vi "Get My Computer Build Spec Children__icon_lib_labview_project_api.vi"(8 "error in (no error)":errorcluster, 11 "Project Reference":refnum<vi>) -> (0 "error out":errorcluster, 2 "Children[]":refnum<vi>[](array[refnum]), 3 "Project Reference Dup":refnum<vi>)   [LabVIEW 2016, in "LabVIEW Project API__icon_lib_labview_project_api.lvlib"]
doc: "Given a Project Path, this VI returns all the Build Spec Children references for the My Computer Target.\n\n<b>Author:</b> JG\n\n<b>ICON Technologies Pty Ltd</b>\nCopyright (C) 1990-2009\nAll Rights Reserved"
uses:
  LabVIEW Project API__icon_lib_labview_project_api.lvlib
panel:
  # "Output"
  # "Input"
  # "ICON Technologies Pty Ltd\nCopyright (C) 1990-2009\nAll Rights Reserved"
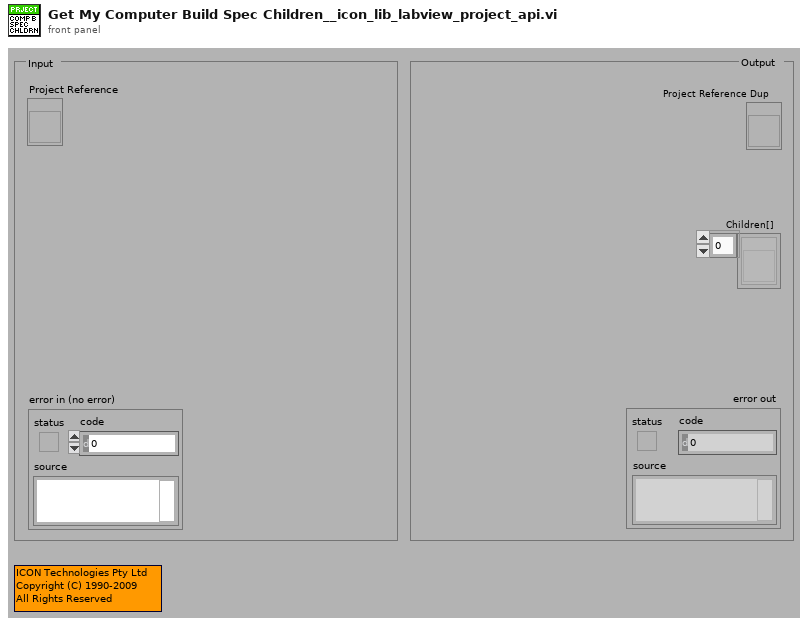
[diagram p1: front panel]
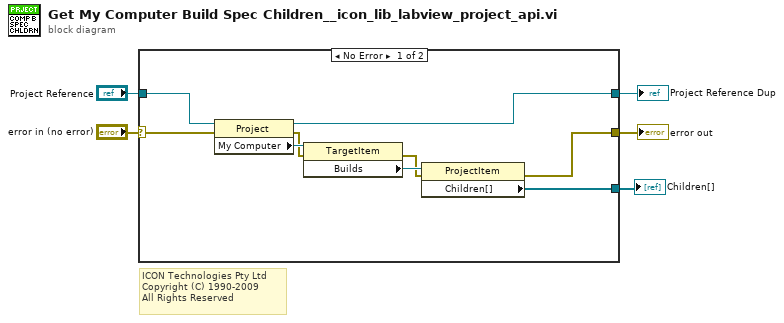
[diagram p0: block diagram]
diagram:
  # "ICON Technologies Pty Ltd\nCopyright (C) 1990-2009\nAll Rights Reserved"
  n1 = case shown="No Error" "error in (no error)" {
    selector: "error in (no error)" -> [w6 w16]
    tunnel: [w8 w16] -> w4
    tunnel: [w10 _] -> w3
    tunnel: [w9 w15] -> w2
    tunnel: "Project Reference" -> [w7 w15]
    frame No Error {
      n2 = property class="Project"(reference=w7, error in=w6) -> (reference out=w9:refnum<vi>, error out=w13:errorcluster, "My Computer"=w14:refnum<vi>)
      n3 = property class="TargetItem"(reference=w14, error in=w13) -> (error out=w11:errorcluster, "Builds"=w12:refnum<vi>)  [unwired: 1 out]
      n4 = property class="ProjectItem"(reference=w12, error in=w11) -> (error out=w8:errorcluster, "Children[]"=w10:refnum<vi>[])  [unwired: 1 out]
    }
    frame Error {
    }
  }
  "error out" <- w4
  "Children[]" <- w3
  "Project Reference Dup" <- w2
